vi "Engine Out - MPCR (Sync Pump).vi"(4 "Control Inputs":T3={"Engine Speed [RPM]"=0.0, "Engine Status"=enum."STALLED", "Load Control \nMode"=enum."Max Speed Governor", "dt(s)"=0.0, "Number of Cylinders"=0, "Engine Displacement [cc]"=0.0, "StoichAFR"=0.0, "Q.LHV Fuel [kJ/kg]"=0.0, "BattV PSU [V]"=0.0, "12V PSU [V]"=0.0, "5V PSU [V]"=0.0, "Pedal Position [%]"=0.0, "Oil Pressure [kPa]"=0.0, "Oil Temp [C]"=0.0, "Oil Level [%]"=0.0, "Engine Coolant Temp (ECT) [C]"=0.0, "Engine Coolant Pressure [kPa]"=0.0, "Rail Pressure [bar]"=0.0, "Fuel Pressure [kPa]"=0.0, "Fuel Temp [C]"=0.0, "Vacuum Pressure [kPa]"=0.0, "Throttle Position [%]"=0.0, "Cam1 Advance [CAD]"=0.0, "Cam2 Advance [CAD]"=0.0, "Cam3 Advance [CAD]"=0.0, "Cam4 Advance [CAD]"=0.0, "CA50 Control Output [CAD]"=[], "CA50 Control Output Valid"=[], "Intake Air Temp (IAT) [C]"=0.0, "Barometric Air Pressure [kPa]"=0.0, "Intake Air Rel. Humidity [%]"=0.0, "Mass Air Flow (MAF) [kg/hr]"=0.0, "Turbo Inlet Air Pressure [kPa]"=0.0, "Turbo Inlet Air Temp [C]"=0.0, "Turbo Outlet Air Pressure [kPa]"=0.0, "Turbo Outlet Air Temp [C]"=0.0, "CAC Outlet Pressure [kPa]"=0.0, "CAC Outlet Temp [C]"=0.0, "Intake Manifold Pressure (MAP) [kPa]"=0.0, "Intake Manifold Temp (MAT) [C]"=0.0, "Exhaust Manifold Pressure [kPa]"=0.0, "Exhaust Manifold Temp [C]"=0.0, "HighP EGR Cooler Outlet Pressure [kPa]"=0.0, "HighP EGR Cooler Outlet Temp [C]"=0.0, "HighP EGR Differential Pressure [kPa]"=0.0, "HighP EGR Valve Position [%]"=0.0, "Turbo Outlet Exhaust Pressure [kPa]"=0.0, "Turbo Outlet Exhaust Temp [C]"=0.0, "VGT Position 1 [%]"=0.0, "VGT Position 2 [%]"=0.0, "Turbo Speed 1 [RPM]"=0.0, "Turbo Speed 2 [RPM]"=0.0, "LowP EGR Differential Pressure [kPa]"=0.0, "LowP EGR Valve Position [%]"=0.0, "UEGO1Lambda"=0.0, "UEGO1_Hot"=FALSE, "UEGO2Lambda"=0.0, "UEGO2_Hot"=FALSE, "Knock Intensity"=[], "Knock"=[]} {"Knock Intensity" format="%.2f"; "CA50 Control Output [CAD]" format="%.2f"; "Exhaust Manifold Temp [C]" format="%#_6f"; "UEGO2Lambda" format="%.2f"; "Intake Manifold Temp (MAT) [C]" format="%#_6f"; "UEGO1Lambda" format="%.2f"}, 5 "Injection Quantities [mg/inj]":T1[](array[typedef]), 6 "Rail Pressure Setpoint [bar]":sgl, 7 "Cam Advance [CAD]":sgl) -> (2 "SyncPump Injections  3&4 (DIx-2)":T2, 3 "SyncPump Injections  1&2 (DIx-1)":T2)   [LabVIEW 2015, in "ECS-RT.lvlib"]
uses:
  ECS-RT.lvlib
  Typedefs/Control Inputs/Control Inputs.ctl
  Typedefs/EPT/Engine Status.ctl
  Typedefs/MISC/Load Control Mode.ctl
  Typedefs/Raw Outputs/DI.ctl
  Typedefs/Control Outputs/Injection Quantity.ctl
  ECS-Shared.lvlib
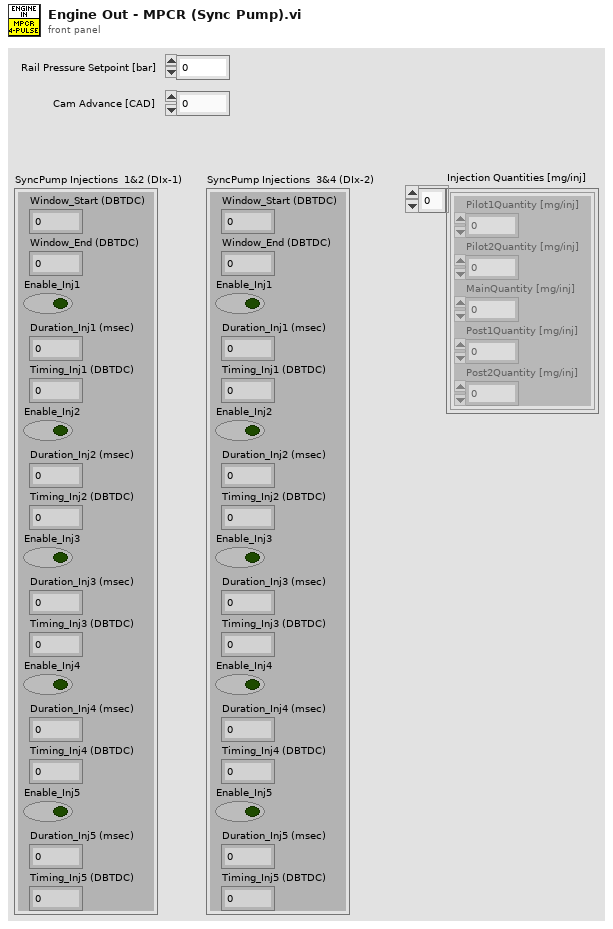
[diagram p1: front panel]
types:
  T1 = typedef "ECS-Shared.lvlib/Injection Quantity.ctl" = cluster{"Pilot1Quantity [mg/inj]":sgl, "Pilot2Quantity [mg/inj]":sgl, "MainQuantity [mg/inj]":sgl, "Post1Quantity [mg/inj]":sgl, "Post2Quantity [mg/inj]":sgl}
  T2 = typedef "ECS-Shared.lvlib/DI.ctl" = cluster{"Window_Start (DBTDC)":sgl, "Window_End (DBTDC)":sgl, "Enable_Inj1":bool, "Duration_Inj1 (msec)":sgl, "Timing_Inj1 (DBTDC)":sgl, "Enable_Inj2":bool, "Duration_Inj2 (msec)":sgl, "Timing_Inj2 (DBTDC)":sgl, "Enable_Inj3":bool, "Duration_Inj3 (msec)":sgl, "Timing_Inj3 (DBTDC)":sgl, "Enable_Inj4":bool, "Duration_Inj4 (msec)":sgl, "Timing_Inj4 (DBTDC)":sgl, "Enable_Inj5":bool, "Duration_Inj5 (msec)":sgl, "Timing_Inj5 (DBTDC)":sgl}
  T3 = typedef "ECS-Shared.lvlib/Control Inputs.ctl" = cluster{"Engine Speed [RPM]":sgl, "Engine Status":T4, "Load Control \nMode":T5, "dt(s)":sgl, "Number of Cylinders":u8, "Engine Displacement [cc]":sgl, "StoichAFR":sgl, "Q.LHV Fuel [kJ/kg]":sgl, "BattV PSU [V]":sgl, "12V PSU [V]":sgl, "5V PSU [V]":sgl, "Pedal Position [%]":sgl, "Oil Pressure [kPa]":sgl, "Oil Temp [C]":sgl, "Oil Level [%]":sgl, "Engine Coolant Temp (ECT) [C]":sgl, "Engine Coolant Pressure [kPa]":sgl, "Rail Pressure [bar]":sgl, "Fuel Pressure [kPa]":sgl, "Fuel Temp [C]":sgl, "Vacuum Pressure [kPa]":sgl, "Throttle Position [%]":sgl, "Cam1 Advance [CAD]":sgl, "Cam2 Advance [CAD]":sgl, "Cam3 Advance [CAD]":sgl, "Cam4 Advance [CAD]":sgl, "CA50 Control Output [CAD]":sgl[], "CA50 Control Output Valid":bool[], "Intake Air Temp (IAT) [C]":sgl, "Barometric Air Pressure [kPa]":sgl, "Intake Air Rel. Humidity [%]":sgl, "Mass Air Flow (MAF) [kg/hr]":sgl, "Turbo Inlet Air Pressure [kPa]":sgl, "Turbo Inlet Air Temp [C]":sgl, "Turbo Outlet Air Pressure [kPa]":sgl, "Turbo Outlet Air Temp [C]":sgl, "CAC Outlet Pressure [kPa]":sgl, "CAC Outlet Temp [C]":sgl, "Intake Manifold Pressure (MAP) [kPa]":sgl, "Intake Manifold Temp (MAT) [C]":sgl, "Exhaust Manifold Pressure [kPa]":sgl, "Exhaust Manifold Temp [C]":sgl, "HighP EGR Cooler Outlet Pressure [kPa]":sgl, "HighP EGR Cooler Outlet Temp [C]":sgl, "HighP EGR Differential Pressure [kPa]":sgl, "HighP EGR Valve Position [%]":sgl, "Turbo Outlet Exhaust Pressure [kPa]":sgl, "Turbo Outlet Exhaust Temp [C]":sgl, "VGT Position 1 [%]":sgl, "VGT Position 2 [%]":sgl, "Turbo Speed 1 [RPM]":sgl, "Turbo Speed 2 [RPM]":sgl, "LowP EGR Differential Pressure [kPa]":sgl, "LowP EGR Valve Position [%]":sgl, "UEGO1Lambda":sgl, "UEGO1_Hot":bool, "UEGO2Lambda":sgl, "UEGO2_Hot":bool, "Knock Intensity":sgl[], "Knock":bool[]}
  T4 = typedef "ECS-Shared.lvlib/Engine Status.ctl" = enum16{"OFF", "STALLED", "CRANKING", "RUNNING", "ACCEL", "DECEL", "SAFE"}
  T5 = typedef "ECS-Shared.lvlib/Load Control Mode.ctl" = enum16{"No Governor", "Min Speed Governor", "Max Speed Governor"}
  T6 = cluster{"PID_Kp":sgl, "PID_Ti":sgl, "PID_Td":sgl, "PID_FF":sgl, "Non-PID_FF":sgl, "PID_Min":sgl, "PID_Max":sgl}
  T7 = cluster{"Min Duration":sgl, "Manual Duration":sgl, "Max Duration":sgl, "Duration Override":bool}
  T8 = cluster{"DBTDC_FQV_Duration":sgl, "PID_Output":sgl}
  T9 = cluster{"ProportionalAction":sgl, "IntegralAction":sgl, "DerivativeAction":sgl}
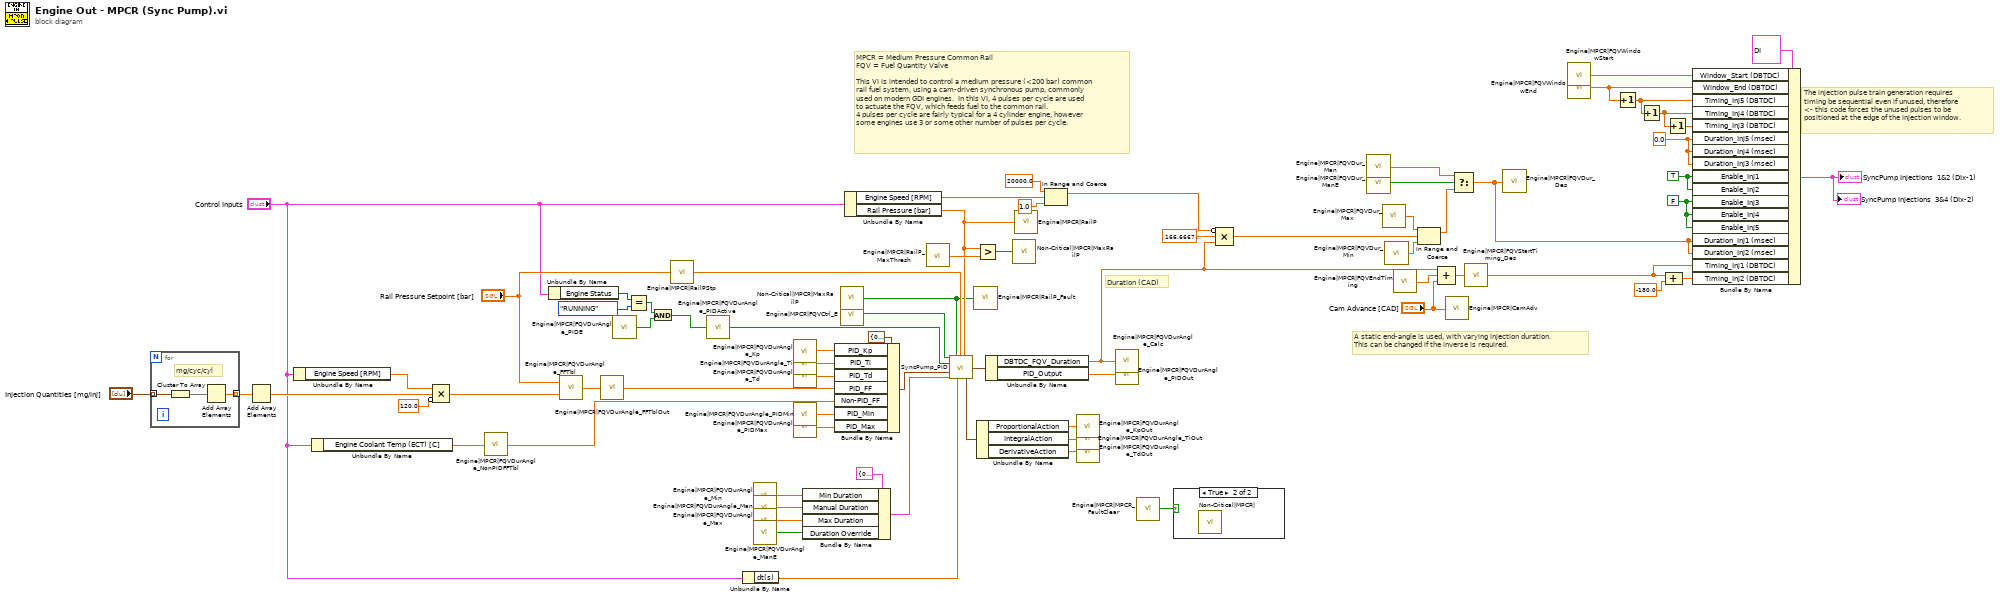
[diagram p0: block diagram]
diagram:
  w41 = sgl 0.0 ("Duration_Inj5 (msec)")
  w48 = FALSE ("Enable_Inj2")
  w42 = TRUE ("Enable_Inj1")
  # "A static end-angle is used, with varying injection duration.  \nThis can be changed if the inverse is required."
  # "MPCR = Medium Pressure Common Rail\nFQV = Fuel Quantity Valve\n\nThis VI is intended to control a medium pressure (<200 bar) common\nrail fuel system, using a cam-driven synchronous pump, commonly\nused on modern GDI engines.  In this VI, 4 pulses per cycle are used\nto actuate the FQV, which feeds fuel to the common rail.  \n4 pulses per cycle are fairly typical for a 4 cylinder engine, however \nsome engines use 3 or some other number of pulses per cycle."
  # "Duration (CAD)"
  # "The injection pulse train generation requires\ntiming be sequential even if unused, therefore \n<- this code forces the unused pulses to be \npositioned at the edge of the injection window."
  n1 = for {
    tunnel: "Injection Quantities [mg/inj]" -> [w73] mode=indexing
    tunnel: [w71] -> w10 mode=indexing
    # "mg/cyc/cyl"
    n2 = Cluster To Array(cluster=w73) -> (array=w72:sgl[])
    n3 = Add Array Elements(numeric array=w72) -> (sum=w71:sgl)
  }
  n4 = Add Array Elements(numeric array=w10) -> (sum=w9:sgl)
  n5 = Unbundle By Name("Control Inputs") -> ("Engine Speed [RPM]"=w20:sgl)
  n6 = Unbundle By Name("Control Inputs") -> ("Engine Coolant Temp (ECT) [C]"=w2:sgl)
  n7 = Compound Arithmetic op=MULTIPLY(w20, w9, invert sgl 120.0 ("value")) -> (w22:sgl)
  n8 = call "Engine|MPCR|FQVDurAngle_NonPIDFFTbl"("X Index"=w2) -> ("Y"=w1:sgl)
  n9 = Unbundle By Name("Control Inputs") -> ("Engine Status"=w8:T4)
  n10 = call "Engine|MPCR|FQVDurAngle_FFTbl"("Y Index"=w22, "X Index"="Rail Pressure Setpoint [bar]") -> ("Z"=w49:sgl)
  n11 = call "Engine|MPCR|FQVDurAngle_FFTblOut"("Value"=w49) -> ()
  n12 = call "Engine|MPCR|FQVDurAngle_PIDE"() -> ("Value"=w5:bool)
  n13 = Equal?(x=w8, y=Engine_Status."RUNNING") -> (x = y?=w6:bool)
  n14 = And(x=w6, y=w5) -> (x .and. y?=w4:bool)
  n15 = call "Engine|MPCR|RailPStp"("Value"="Rail Pressure Setpoint [bar]") -> ()
  n16 = call "Engine|MPCR|FQVDurAngle_PIDActive"("Value"=w4) -> ()
  n17 = Unbundle By Name("Control Inputs") -> ("dt(s)"=w54:sgl)
  n18 = call "Engine|MPCR|FQVDurAngle_Min"() -> ("Value"=w65:sgl)
  n19 = call "Engine|MPCR|FQVDurAngle_Man"() -> ("Value"=w66:sgl)
  n20 = call "Engine|MPCR|FQVDurAngle_Max"() -> ("Value"=w64:sgl)
  n21 = call "Engine|MPCR|FQVDurAngle_ManE"() -> ("Value"=w63:bool)
  n22 = call "Engine|MPCR|FQVDurAngle_Kp"() -> ("Value"=w58:sgl)
  n23 = call "Engine|MPCR|FQVDurAngle_Ti"() -> ("Value"=w59:sgl)
  n24 = call "Engine|MPCR|FQVDurAngle_Td"() -> ("Value"=w60:sgl)
  n25 = call "Engine|MPCR|FQVDurAngle_PIDMin"() -> ("Value"=w61:sgl)
  n26 = call "Engine|MPCR|FQVDurAngle_PIDMax"() -> ("Value"=w62:sgl)
  n27 = Bundle By Name(cluster=T7 {"Min Duration"=0.0, "Manual Duration"=0.0, "Max Duration"=0.0, "Duration Override"=FALSE} ("Output Management Controls"), "Min Duration"=w65, "Manual Duration"=w66, "Max Duration"=w64, "Duration Override"=w63) -> (w52:T7)
  n28 = Bundle By Name(cluster=T6 {"PID_Kp"=0.0, "PID_Ti"=0.01, "PID_Td"=0.0, "PID_FF"=0.0, "Non-PID_FF"=0.0, "PID_Min"=-100.0, "PID_Max"=100.0} ("PID Settings"), "PID_Kp"=w58, "PID_Ti"=w59, "PID_Td"=w60, "PID_FF"=w49, "Non-PID_FF"=w1, "PID_Min"=w61, "PID_Max"=w62) -> (w12:T6)
  n29 = call "Non-Critical|MPCR|MaxRailP"() -> ("Fault"=w14:bool)  [unwired: 2 in]
  n30 = call "Engine|MPCR|FQVCtrl_E"() -> ("Value"=w53:bool)
  n31 = Unbundle By Name("Control Inputs") -> ("Engine Speed [RPM]"=w25:sgl, "Rail Pressure [bar]"=w16:sgl)
  n32 = call "Engine|MPCR|RailP_MaxThresh"() -> ("Value"=w39:sgl)
  n33 = call "SyncPump_PID.vi"("Control Enable"=w53, "Fault Input"=w14, "Rail Press Setpoint"="Rail Pressure Setpoint [bar]", "Rail Pressure"=w16, "PID Enable"=w4, "PID Settings"=w12, "Output Management Controls"=w52, "dt (s)"=w54) -> ("Output"=w51:T8, "PID_Action_Output"=w50:T9)  [unwired: 6 in]
  n34 = call "Engine|MPCR|RailP_Fault"("Value"=w14) -> ()
  n35 = Greater?(x=w16, y=w39) -> (0:w19:bool)
  n36 = Unbundle By Name(w50) -> ("ProportionalAction"=w69:sgl, "IntegralAction"=w68:sgl, "DerivativeAction"=w67:sgl)
  n37 = Unbundle By Name(w51) -> ("DBTDC_FQV_Duration"=w37:sgl, "PID_Output"=w56:sgl)
  n38 = call "Non-Critical|MPCR|MaxRailP"("Fault"=w19) -> ()  [unwired: 2 in]
  n39 = call "Engine|MPCR|RailP"("Value"=w16) -> ()
  n40 = In Range and Coerce(upper limit=20000.0, x=w25, lower limit=1.0) -> (coerced(x)=w24:dbl)  [unwired: 1 out]
  n41 = call "Engine|MPCR|FQVDurAngle_KpOut"("Value"=w69) -> ()
  n42 = call "Engine|MPCR|FQVDurAngle_TiOut"("Value"=w68) -> ()
  n43 = call "Engine|MPCR|FQVDurAngle_TdOut"("Value"=w67) -> ()
  n44 = call "Engine|MPCR|FQVDurAngle_Calc"("Value"=w37) -> ()
  n45 = call "Engine|MPCR|FQVDurAngle_PIDOut"("Value"=w56) -> ()
  n46 = call "Engine|MPCR|MPCR_FaultClear"() -> ("Value"=w70:bool)
  n47 = case shown="True" w70 {
    frame False {
    }
    frame True {
      n48 = call "Non-Critical|MPCR|"() -> ()  [unwired: 3 in]
    }
  }
  n49 = Compound Arithmetic op=MULTIPLY(invert w24, sgl 166.6667 ("value"), w37) -> (w30:dbl)
  n50 = call "Engine|MPCR|FQVDur_Man"() -> ("Value"=w57:sgl)
  n51 = call "Engine|MPCR|FQVDur_ManE"() -> ("Value"=w55:bool)
  n52 = call "Engine|MPCR|FQVDur_Max"() -> ("Value"=w29:sgl)
  n53 = call "Engine|MPCR|FQVDur_Min"() -> ("Value"=w28:sgl)
  n54 = call "Engine|MPCR|FQVEndTiming"() -> ("Value"=w36:sgl)
  n55 = In Range and Coerce(upper limit=w29, x=w30, lower limit=w28) -> (coerced(x)=w31:dbl)  [unwired: 1 out]
  n56 = Compound Arithmetic op=ADD(w37, w36, "Cam Advance [CAD]") -> (w23:sgl)
  n57 = call "Engine|MPCR|CamAdv"("Value"="Cam Advance [CAD]") -> ()
  n58 = Select(t=w57, s=w55, f=w31) -> (s? t:f=w32:dbl)
  n59 = call "Engine|MPCR|FQVStartTiming_Des"("Value"=w23) -> ()
  n60 = call "Engine|MPCR|FQVDur_Des"("Value"=w32) -> ()
  n61 = call "Engine|MPCR|FQVWindowStart"() -> ("Value"=w47:sgl)
  n62 = call "Engine|MPCR|FQVWindowEnd"() -> ("Value"=w46:sgl)
  n63 = Increment(x=w46) -> (x+1=w43:sgl)
  n64 = Increment(x=w43) -> (x+1=w44:sgl)
  n65 = Compound Arithmetic op=ADD(w23, sgl -180.0 ("y")) -> (w34:sgl)
  n66 = Increment(x=w44) -> (x+1=w45:sgl)
  n67 = Bundle By Name(cluster=T2 {"Window_Start (DBTDC)"=0.0, "Window_End (DBTDC)"=0.0, "Enable_Inj1"=FALSE, "Duration_Inj1 (msec)"=0.0, "Timing_Inj1 (DBTDC)"=0.0, "Enable_Inj2"=FALSE, "Duration_Inj2 (msec)"=0.0, "Timing_Inj2 (DBTDC)"=0.0, "Enable_Inj3"=FALSE, "Duration_Inj3 (msec)"=0.0, "Timing_Inj3 (DBTDC)"=0.0, "Enable_Inj4"=FALSE, "Duration_Inj4 (msec)"=0.0, "Timing_Inj4 (DBTDC)"=0.0, "Enable_Inj5"=FALSE, "Duration_Inj5 (msec)"=0.0, "Timing_Inj5 (DBTDC)"=0.0} ("SP-Inj"), "Window_Start (DBTDC)"=w47, "Window_End (DBTDC)"=w46, "Timing_Inj5 (DBTDC)"=w43, "Timing_Inj4 (DBTDC)"=w44, "Timing_Inj3 (DBTDC)"=w45, "Duration_Inj5 (msec)"=w41, "Duration_Inj4 (msec)"=w41, "Duration_Inj3 (msec)"=w41, "Enable_Inj1"=w42, "Enable_Inj2"=w42, "Enable_Inj3"=w48, "Enable_Inj4"=w48, "Enable_Inj5"=w48, "Duration_Inj1 (msec)"=w32, "Duration_Inj2 (msec)"=w32, "Timing_Inj1 (DBTDC)"=w23, "Timing_Inj2 (DBTDC)"=w34) -> (→"SyncPump Injections  1&2 (DIx-1)" →"SyncPump Injections  3&4 (DIx-2)":T2)
